vi "readCRC.vi"(8 "error in (no error)":errorcluster, 11 "ModbusBuffer in":refnum<class "ModbusBuffer.lvclass">) -> (0 "error out":errorcluster, 2 "Output":u16, 3 "ModbusBuffer out":refnum<class "ModbusBuffer.lvclass">)   [LabVIEW 2016, in "RTModbus.lvlib" / "ModbusBuffer.lvclass"]
uses:
  ModbusBuffer.lvclass
  ModbusBuffer.lvclass/ModbusBuffer.ctl
  readInstructionByte.vi
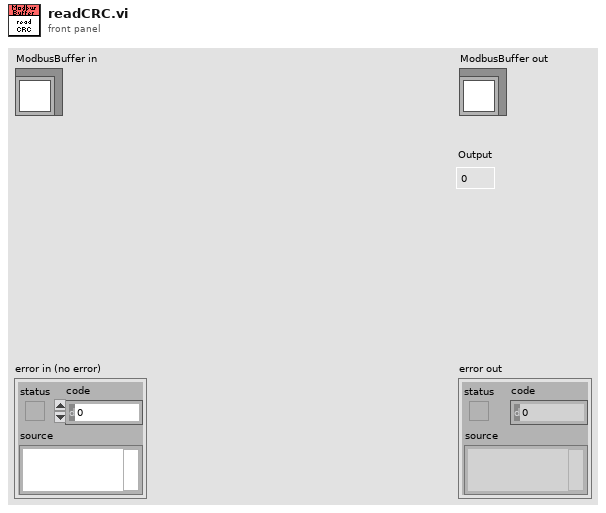
[diagram p1: front panel]
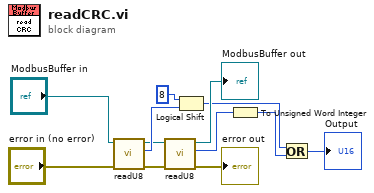
[diagram p0: block diagram]
diagram:
  n1 = call "readU8.vi"("error in (no error)"="error in (no error)", "ModbusBuffer in"="ModbusBuffer in") -> ("error out"=w2:errorcluster, "Output"=w11:u8, "ModbusBuffer out"=w8:refnum<class "ModbusBuffer.lvclass">)  [unwired: 7 in]
  n2 = call "readU8.vi"("error in (no error)"=w2, "ModbusBuffer in"=w8) -> ("error out"=→"error out":errorcluster, "Output"=w12:u8, "ModbusBuffer out"=→"ModbusBuffer out":refnum<class "ModbusBuffer.lvclass">)  [unwired: 7 in]
  n3 = Logical Shift(y=i16 8, x=w11) -> (x << y=w5:u8)
  n4 = To Unsigned Word Integer(number=w12) -> (unsigned 16bit integer=w6:u16)
  n5 = Or(x=w5, y=w6) -> (x .or. y?=→"Output":u16)
